vi "HEWH Water Cp.vi"(8 "Error In":errorcluster, 11 "Input Temperature (°F)":dbl) -> (0 "Error Out":errorcluster, 3 "Specific Heat (BTU/lbm*F)":dbl)   [LabVIEW 2016]
uses:
  <vilib>/Analysis/NI_AALPro.lvlib
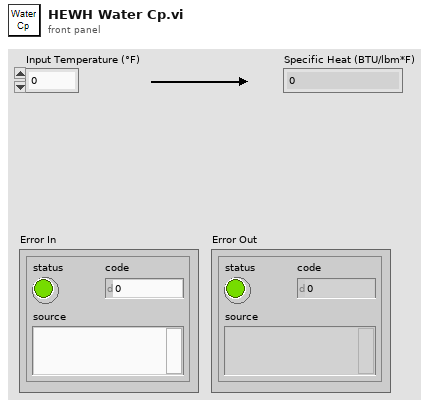
[diagram p1: front panel]
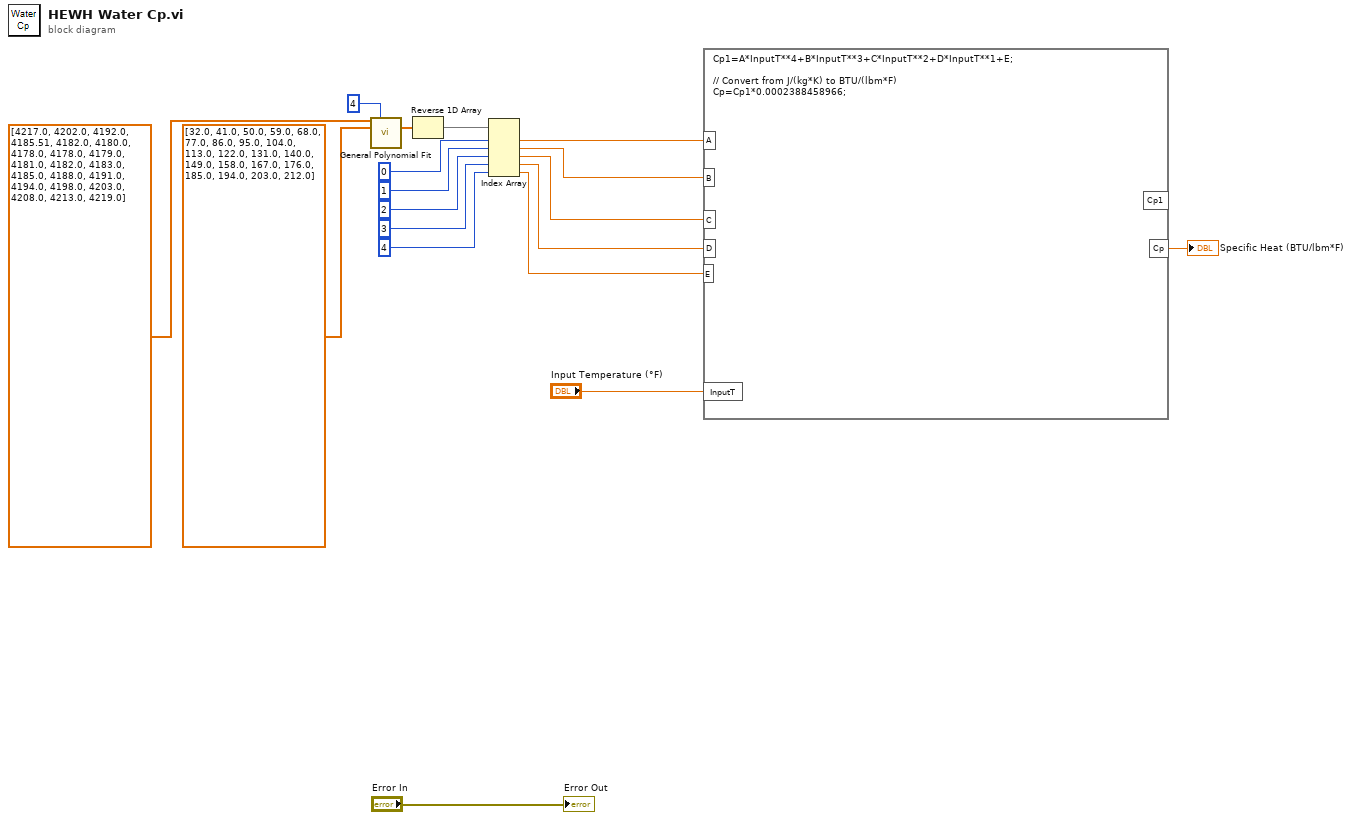
[diagram p0: block diagram]
diagram:
  n1 = call <vilib>:"General Polynomial Fit.vi"("Y"=dbl[] [4217.0, 4202.0, 4192.0, 4185.51, 4182.0, 4180.0, 4178.0, 4178.0, 4179.0, 4181.0, 4182.0, 4183.0, 4185.0, 4188.0, 4191.0, 4194.0, 4198.0, 4203.0, 4208.0, 4213.0, 4219.0], "polynomial order"=4, "X"=dbl[] [32.0, 41.0, 50.0, 59.0, 68.0, 77.0, 86.0, 95.0, 104.0, 113.0, 122.0, 131.0, 140.0, 149.0, 158.0, 167.0, 176.0, 185.0, 194.0, 203.0, 212.0]) -> ("Polynomial Coefficients"=w5:dbl[])  [unwired: 9 in, 3 out]
  n2 = Reverse 1D Array(array=w5) -> (reversed array=w6:dbl[])
  n3 = Index Array(array=w6, index #1=0 ("index"), index #2=1 ("index"), index #3=2 ("index"), index #4=3 ("index"), index #5=4 ("index")) -> (element #1=w11:dbl, element #2=w12:dbl, element #3=w13:dbl, element #4=w14:dbl, element #5=w16:dbl)
  n4 = formula code="Cp1=A*InputT**4+B*InputT**3+C*InputT**2+D*InputT**1+E;\n\n// Convert from J/(kg*K) to BTU/(lbm*F)\nCp=Cp1*0.0002388458966;"("A"=w11, "B"=w12, "C"=w13, "D"=w14, "InputT"="Input Temperature (°F)", "E"=w16) -> ("Cp"=→"Specific Heat (BTU/lbm*F)":dbl)  [unwired: 1 out]
  "Error Out" <- "Error In"
